vi "Day05-01_글로벌 변수(FGV) 열거형 상수.vi"(9 "숫자형":dbl, 10 "열거형":enum16{"뺄셈", "덧셈", "입력"}(ring)) -> (1 "결과값":dbl)   [LabVIEW 2021]
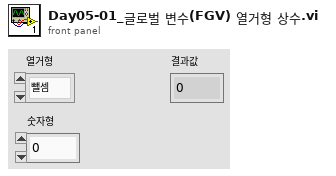
[diagram p1: front panel]
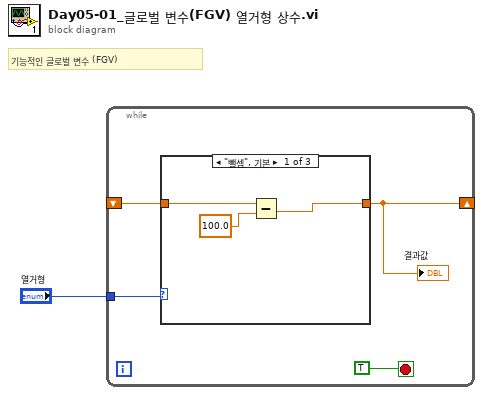
[diagram p0: block diagram]
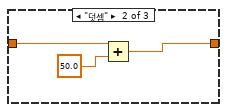
[diagram p2: hidden frame]
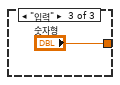
[diagram p3: hidden frame]
diagram:
  # "기능적인 글로벌 변수 (FGV)"
  n1 = while {
    tunnel: "열거형" -> [w5]
    shift-right: [w2] -> _
    shift-left: _ -> [w4]
    stop <- TRUE stop-if-true
    n2 = case shown="\"뺄셈\", 기본" w5 {
      tunnel: w4 -> [w7 w11 _]
      tunnel: [w6 w10 "숫자형"] -> w2
      frame "뺄셈", Default {
        n3 = Subtract(x=w7, y=100.0) -> (x-y=w6:dbl)
      }
      frame "덧셈" {
        n4 = Add(x=w11, y=50.0) -> (x+y=w10:dbl)
      }
      frame "입력" {
      }
    }
    "결과값" <- w2
  }
